vi "hbEnable_data_v2.vi"(11 "file path 2":path=path "C:/luminartech/ManufacturingTools/TS_Automation/Programs/Labview/bring_up/hbEnable/hbEnable_resp.txt") -> (0 "HEAT":dbl, 1 "COOL":dbl, 3 "data array":dbl[](array[numeric]))   [LabVIEW 2018]
panel:
  out "PumpTEC_min":dbl
  out "PumpTEC_max":dbl
  out "LaserPower_min":dbl
  out "LaserPower_max":dbl
  out "LaserSeedTemp_min":dbl
  out "LaserSeedTemp_max":dbl
  out "size(s)":i32
  out "text 2":string[](array[string])
  out "line 2":string
  out "data table":dbl[][](array[numeric])
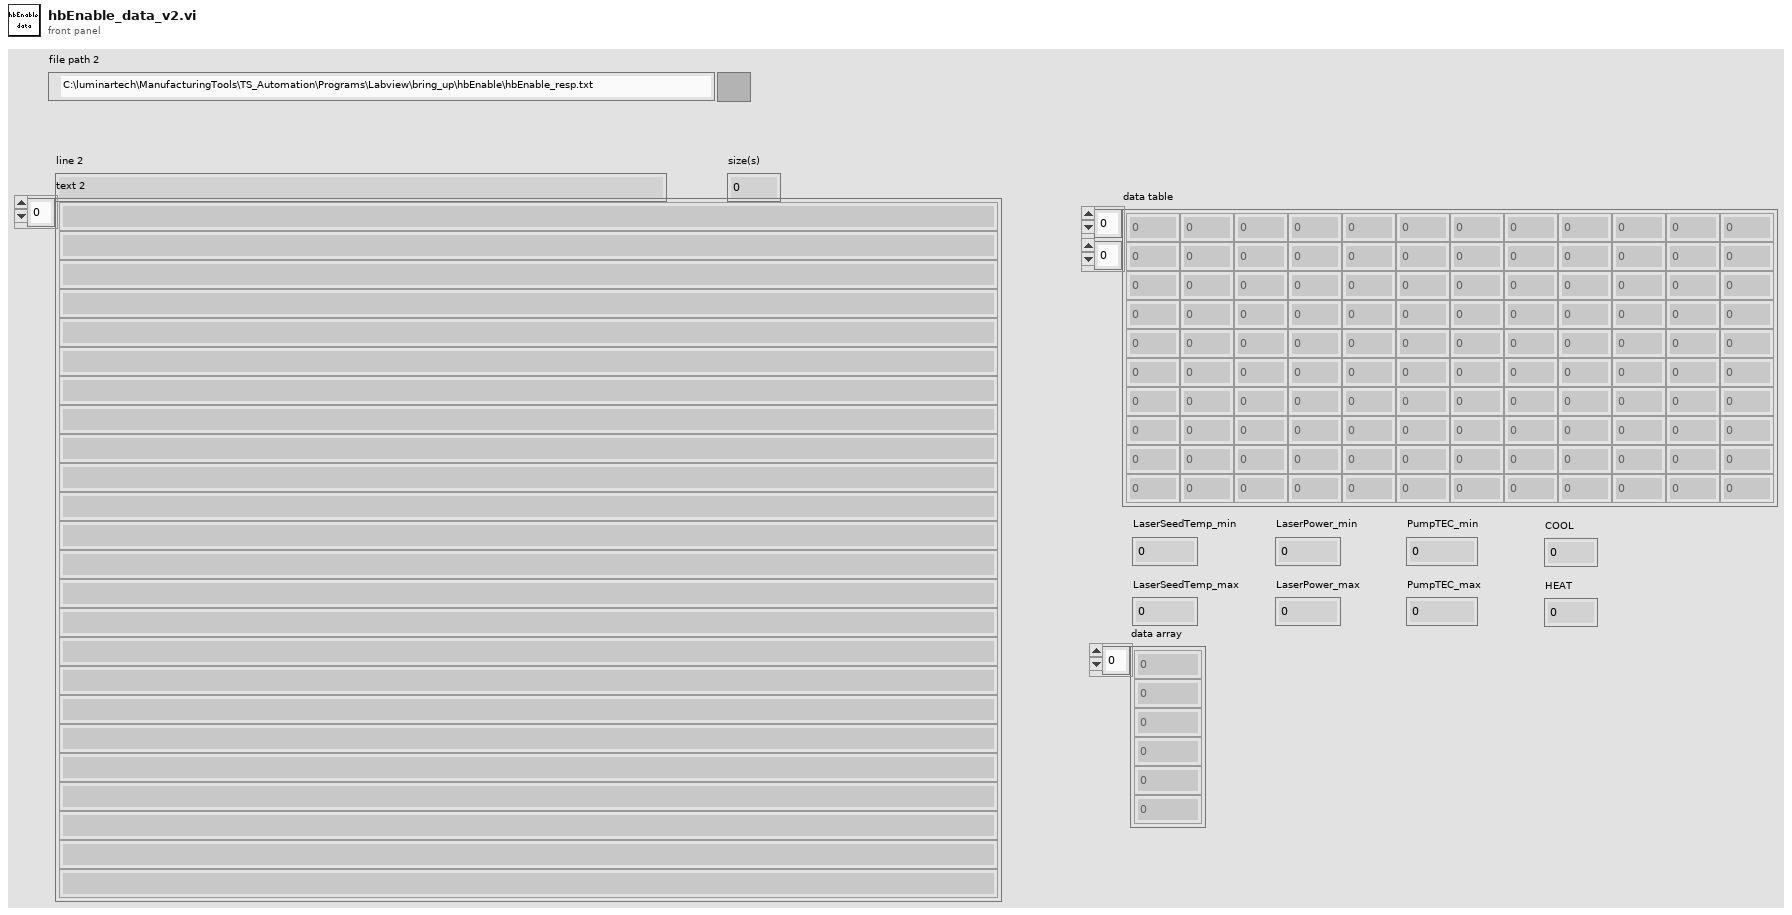
[diagram p1: front panel]
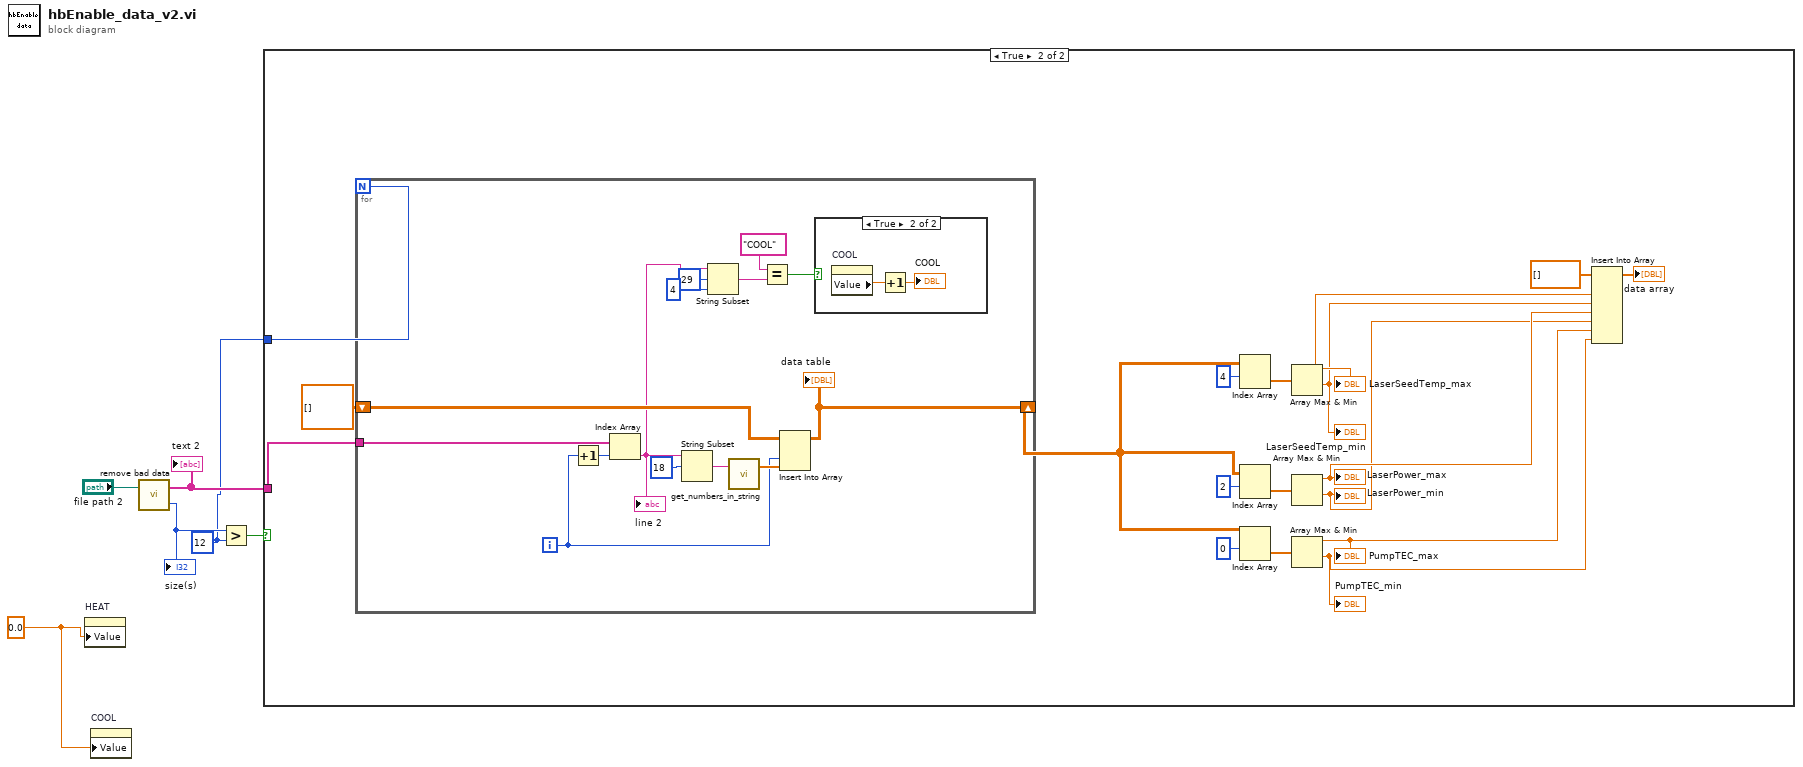
[diagram p0: block diagram]
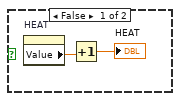
[diagram p3: hidden frame]
diagram:
  w1 = 0.0 ("COOL")
  w2 = 12 ("y")
  n1 = property on="HEAT" class="DigNum (strict)"("Value"=w1) -> ()  [unwired: 2 in, 2 out]
  n2 = property on="COOL" class="DigNum (strict)"("Value"=w1) -> ()  [unwired: 2 in, 2 out]
  n3 = call "remove bad data.vi"("file path"="file path 2") -> ("size(s)"=w3:i32, "text 2"=w4:string[])  [unwired: 1 in]
  "text 2" <- w4
  "size(s)" <- w3
  n4 = Greater?(x=w3, y=w2) -> (0:w5:bool)
  n5 = case shown="True" w5 {
    tunnel: w4 -> [_ w23]
    tunnel: w2 -> [_ w22]
    frame False {
    }
    frame True {
      n6 = for {
        N: w22 -> [_]
        shift-right: [w34] -> w15
        shift-left: dbl[][] [] -> [w35]
        tunnel: w23 -> [w31]
        i -> [w32]
        n7 = Increment(x=w32) -> (x+1=w38:i32)
        n8 = Index Array(array=w31, index=w38) -> (element=w25:string)
        "line 2" <- w25
        n9 = String Subset(string=w25, offset (0)=18) -> (substring=w36:string)  [unwired: 1 in]
        n10 = String Subset(string=w25, offset (0)=29, length (rest)=4 ("length (rest)")) -> (substring=w26:string)
        n11 = call "get_numbers_in_string.vi"("String"=w36) -> ("Extracted Numbers"=w33:dbl[])  [unwired: 1 in, 1 out]
        n12 = Equal?(x="COOL", y=w26) -> (x = y?=w27:bool)
        n13 = Insert Into Array(array=w35, index (col)=w32, new element=w33) -> (w34:dbl[][])  [unwired: 1 in]
        "data table" <- w34
        n14 = case shown="True" w27 {
          frame False {
            n15 = property on="HEAT" class="DigNum (strict)"() -> ("Value"=w40:dbl)  [unwired: 2 in, 2 out]
            n16 = Increment(x=w40) -> (x+1=→"HEAT":dbl)
          }
          frame True {
            n17 = property on="COOL" class="DigNum (strict)"() -> ("Value"=w42:dbl)  [unwired: 2 in, 2 out]
            n18 = Increment(x=w42) -> (x+1=→"COOL":dbl)
          }
        }
      }
      n19 = Index Array(array=w15, index (row)=4) -> (element=w21:dbl[])  [unwired: 1 in]
      n20 = Index Array(array=w15, index (row)=2) -> (element=w19:dbl[])  [unwired: 1 in]
      n21 = Index Array(array=w15, index (row)=0) -> (element=w17:dbl[])  [unwired: 1 in]
      n22 = Array Max & Min(array=w21) -> (max value=w14:dbl, min value=w13:dbl)  [unwired: 2 out]
      "LaserSeedTemp_max" <- w14
      "LaserSeedTemp_min" <- w13
      n23 = Array Max & Min(array=w19) -> (max value=w12:dbl, min value=w11:dbl)  [unwired: 2 out]
      "LaserPower_max" <- w12
      "LaserPower_min" <- w11
      n24 = Array Max & Min(array=w17) -> (max value=w10:dbl, min value=w9:dbl)  [unwired: 2 out]
      "PumpTEC_max" <- w10
      "PumpTEC_min" <- w9
      n25 = Insert Into Array(array=dbl[] [], new element #1=w14, new element #2=w13, new element #3=w12, new element #4=w11, new element #5=w10, new element #6=w9) -> (→"data array":dbl[])  [unwired: 1 in]
    }
  }
